vi "Report Write Graph Data.vi"(8 "error in (no error)":errorcluster, 10 "report in":refnum<class "NI_report.lvclass">, 11 "Hardware Resources in":T1={"Test Setting"={"Test_Num"=0, "Test_ID"=0, "Proc_ID"=0, "Max Force"=0.0, "User"="", "SN"="", "Date"=""}, "Measurements"=[[""]], "LOG REF"=refnum, "Report Template"=path "", "Save Report path"=path "", "Data File Path"=path "", "Popup Dialog"=FALSE}) -> (0 "error out":errorcluster, 2 "report out":refnum<class "NI_report.lvclass">, 3 "Hardware Resources out":T1)   [LabVIEW 2020, in "Report.lvlib"]
doc: "Perform the acquisition. Replace the contents of this diagram with calls to acquisition hardware."
uses:
  Report.lvlib
  REP Configuration.ctl
  Test Setting.ctl
  <vilib>/Utility/NIReport.llb/NI_report.lvclass
  <vilib>/Utility/NIReport.llb/HTML Report Image Alignment.ctl
  <vilib>/Utility/NIReport.llb/NI_ReportGenerationCore.lvlib
panel:
  out "V  Chart 2":dbl[][](graph)
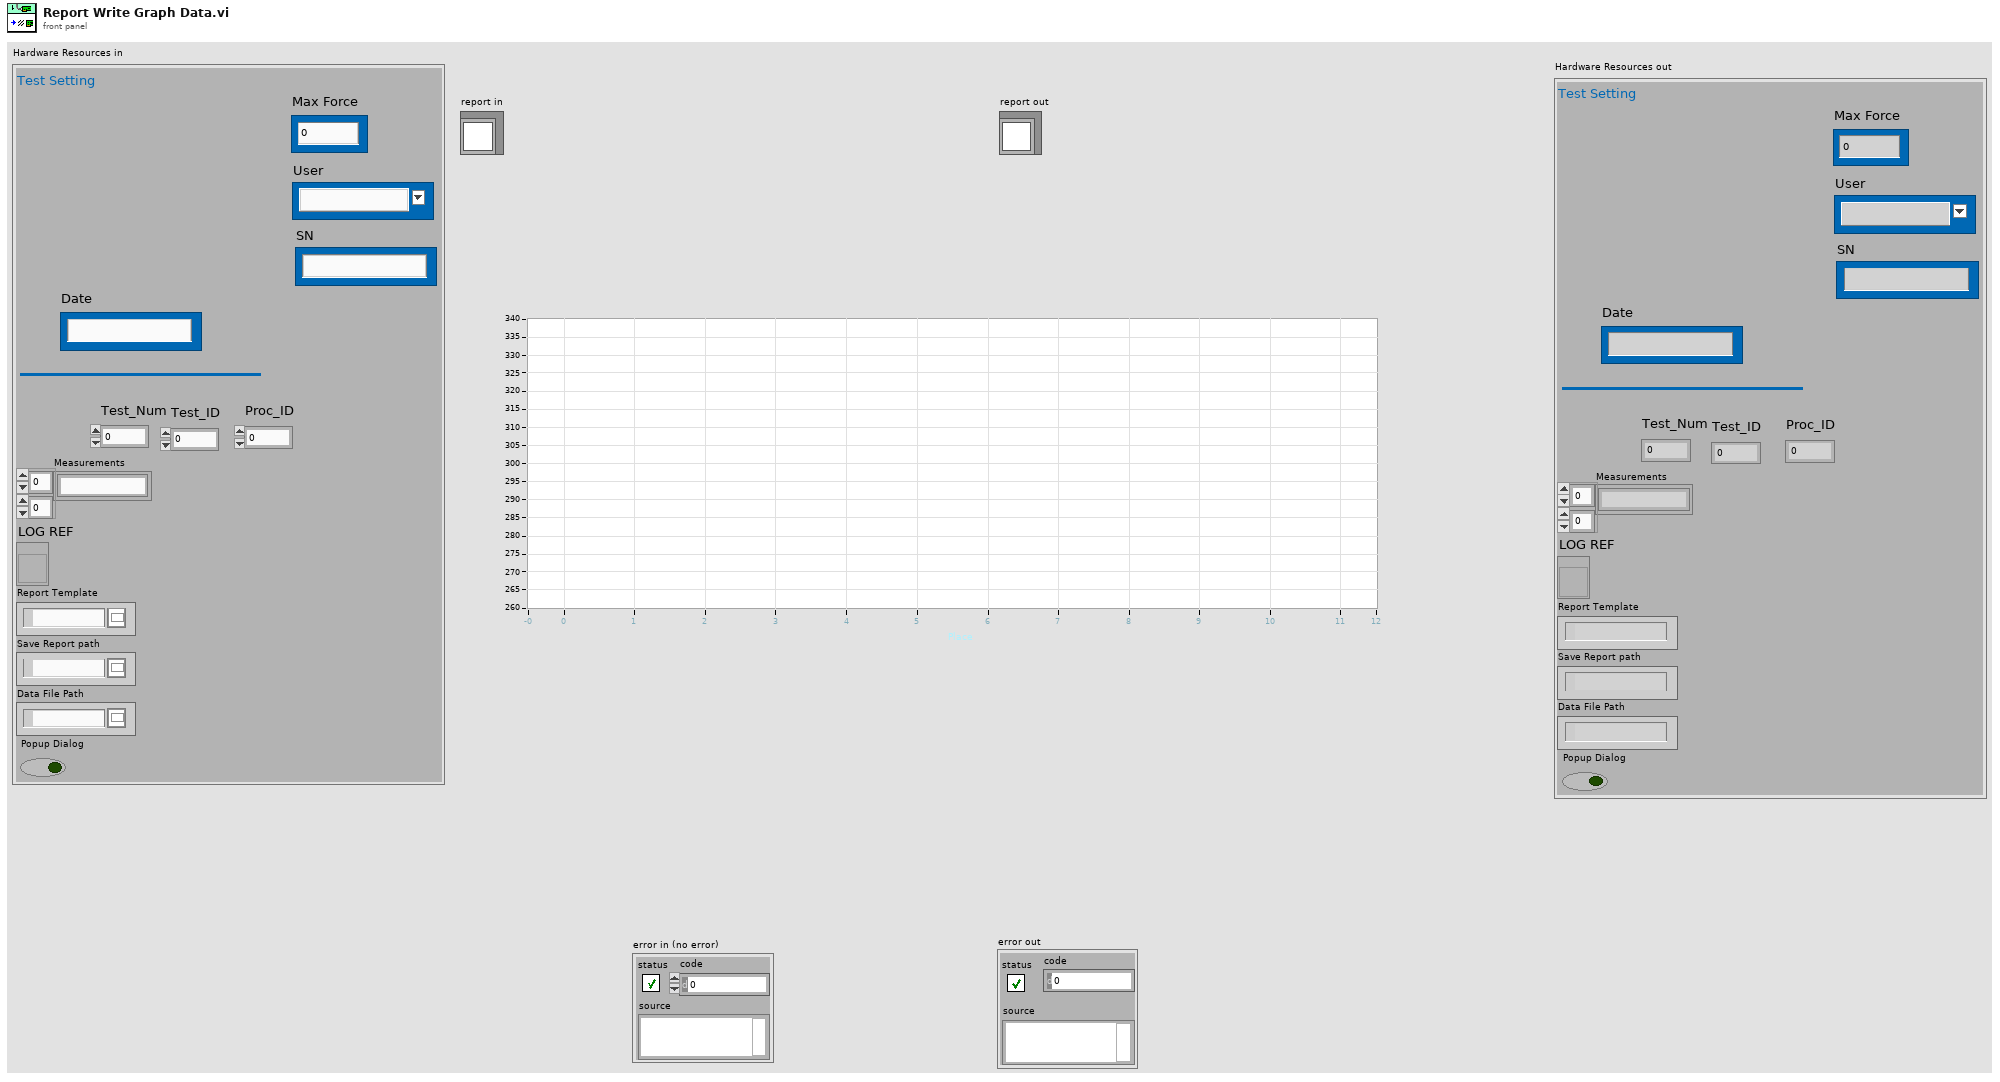
[diagram p1: front panel]
types:
  T1 = typedef "Report.lvlib/REP Configuration.ctl" = cluster{"Test Setting":T2, "Measurements":string[][], "LOG REF":refnum<vi>, "Report Template":path, "Save Report path":path, "Data File Path":path, "Popup Dialog":bool}
  T2 = typedef "Report.lvlib/Test Setting.ctl" = cluster{"Test_Num":i32, "Test_ID":i32, "Proc_ID":i32, "Max Force":dbl, "User":string, "SN":string, "Date":string}
  T3 = cluster{"position (Excel)":cluster{"row":i32, "column":i32}, "name (Excel)":string, "bookmark (Word)":string}
  T4 = typedef "NI_ReportGenerationCore.lvlib/HTML Report Image Alignment.ctl" = enum16{"(default)", "LEFT", "RIGHT", "TOP", "TEXTTOP", "MIDDLE", "ABSMIDDLE", "BASELINE", "BOTTOM", "ABSBOTTOM"}
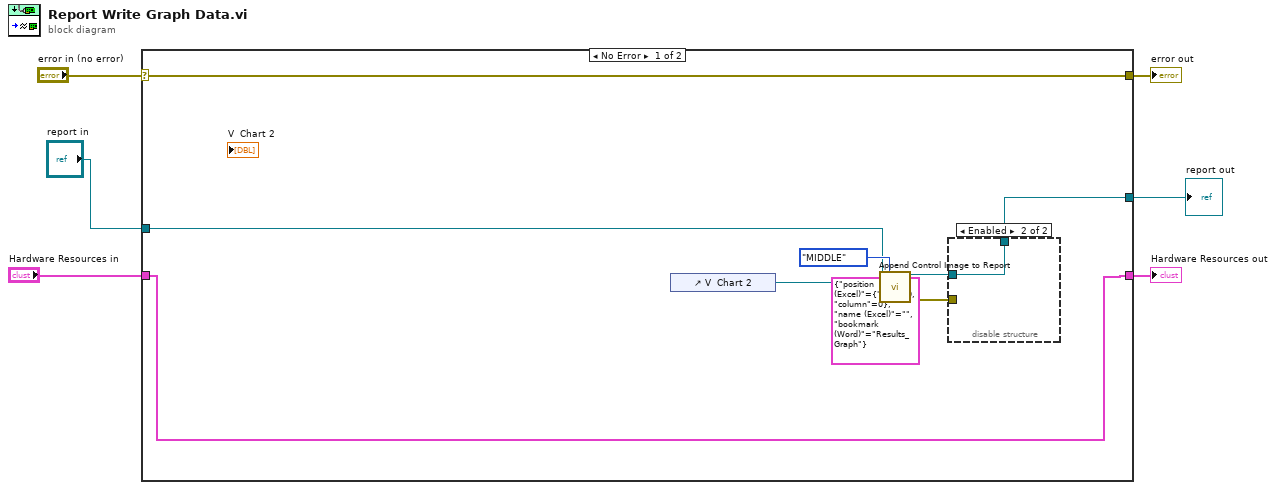
[diagram p0: block diagram]
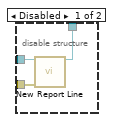
[diagram p2: hidden frame]
diagram:
  n1 = case shown="No Error" "error in (no error)" {
    selector: "error in (no error)" -> [w15 w21]
    tunnel: [w15 w21] -> w5
    tunnel: "Hardware Resources in" -> [w10 w22]
    tunnel: [w10 w22] -> w3
    tunnel: [w9 w20] -> w2
    tunnel: "report in" -> [w8 w20]
    frame No Error {
      n2 = control-ref of="V  Chart 2"() -> (w12:refnum<vi>)
      n3 = call-dynamic "Append Control Image to Report.vi"("report in"=w8, "alignment (default)"=HTML_Report_Image_Alignment."MIDDLE", "ctrl reference"=w12, "MS Office parameters"=T3 {"position (Excel)"={"row"=0, "column"=0}, "name (Excel)"="", "bookmark (Word)"="Results_Graph"}) -> ("report out"=w13:refnum<class "NI_report.lvclass">, "error out"=w11:errorcluster)  [unwired: 8 in, 2 out]
      n4 = disable-structure shown="Enabled" {
        disable-tunnel: w13 -> [w18 w19]
        disable-tunnel: w11 -> [w17 _]
        disable-tunnel: [w16 w19] -> w9
        frame Disabled {
          n5 = call-dynamic "New Report Line.vi"("report in"=w18, "error in (no error)"=w17) -> ("report out"=w16:refnum<class "NI_report.lvclass">)  [unwired: 12 in, 1 out]
        }
        frame Enabled {
        }
      }
    }
    frame Error {
    }
  }
  "Hardware Resources out" <- w3
  "error out" <- w5
  "report out" <- w2
